vi "CSVlog.vi"() -> ()   [LabVIEW 2020]
uses:
  <vilib>/Utility/file.llb/Write Delimited Spreadsheet (string).vi
panel:
  in  "file path (dialog if empty)":path
  in  "Cluster":cluster{"Numeric":dbl, "String":string}
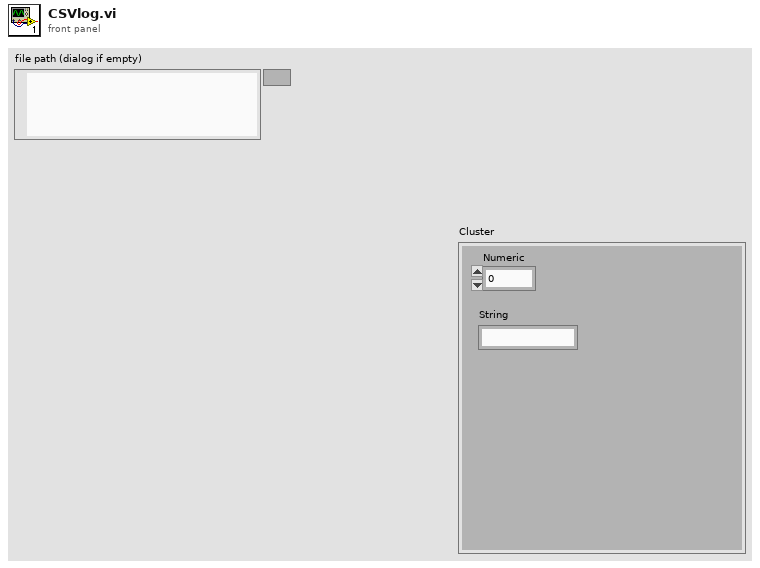
[diagram p1: front panel]
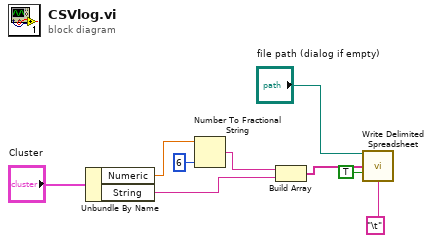
[diagram p0: block diagram]
diagram:
  n1 = Unbundle By Name("Cluster") -> ("Numeric"=w8:dbl, "String"=w5:string)
  n2 = Number To Fractional String(number=w8, precision (6)=i16 6) -> (F-format string=w6:string)  [unwired: 2 in]
  n3 = Build Array(w6, w5) -> (w4:string[])
  n4 = call-poly <vilib>:"Write Delimited Spreadsheet.vi"("file path (dialog if empty)"="file path (dialog if empty)", "1D data"=w4, "append to file? (new file:F)"=TRUE, "delimiter (\\t)"="\t" ("delimiter (\\t)")) -> ()  [unwired: 10 in, 2 out]
